vi "SplineHelp_getQuinticSplinesFromControlVectors_ORIG.vi"(11 "ControlVectors":T1[](array[typedef])) -> (0 "error out":errorcluster, 3 "splines":T2[](array[typedef]))   [LabVIEW 2019]
doc: "Returns a set of quintic splines corresponding to the provided control vectors. The user is free to set the direction of all control vectors. Continuous curvature is guaranteed throughout the path.\n\nParameters:\n - controlVectors - The control vectors.\n\nReturns:\n - Splines - A vector of quintic hermite splines that interpolate through the provided waypoints.\n - Error Out - The returned error cluster"
uses:
  SPLINE.ctl
  <vilib>/Analysis/Matrix/Datatypes/RealMatrix.ctl
  SPLINE_CTRL_VECTOR.ctl
  Trajectory_Library.lvlib
  <vilib>/Analysis/Matrix/NI_Matrix.lvlib
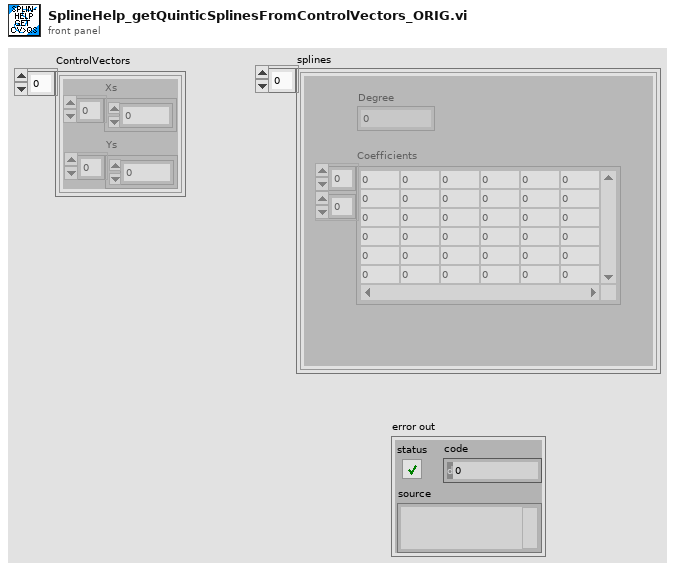
[diagram p1: front panel]
types:
  T1 = typedef "Trajectory_Library.lvlib/SPLINE_CTRL_VECTOR.ctl" = cluster{"Xs":dbl[], "Ys":dbl[]}
  T2 = typedef "Trajectory_Library.lvlib/SPLINE.ctl" = cluster{"Degree":i32, "Coefficients":T3}
  T3 = typedef "NI_Matrix.lvlib/RealMatrix.ctl" = dbl[][]
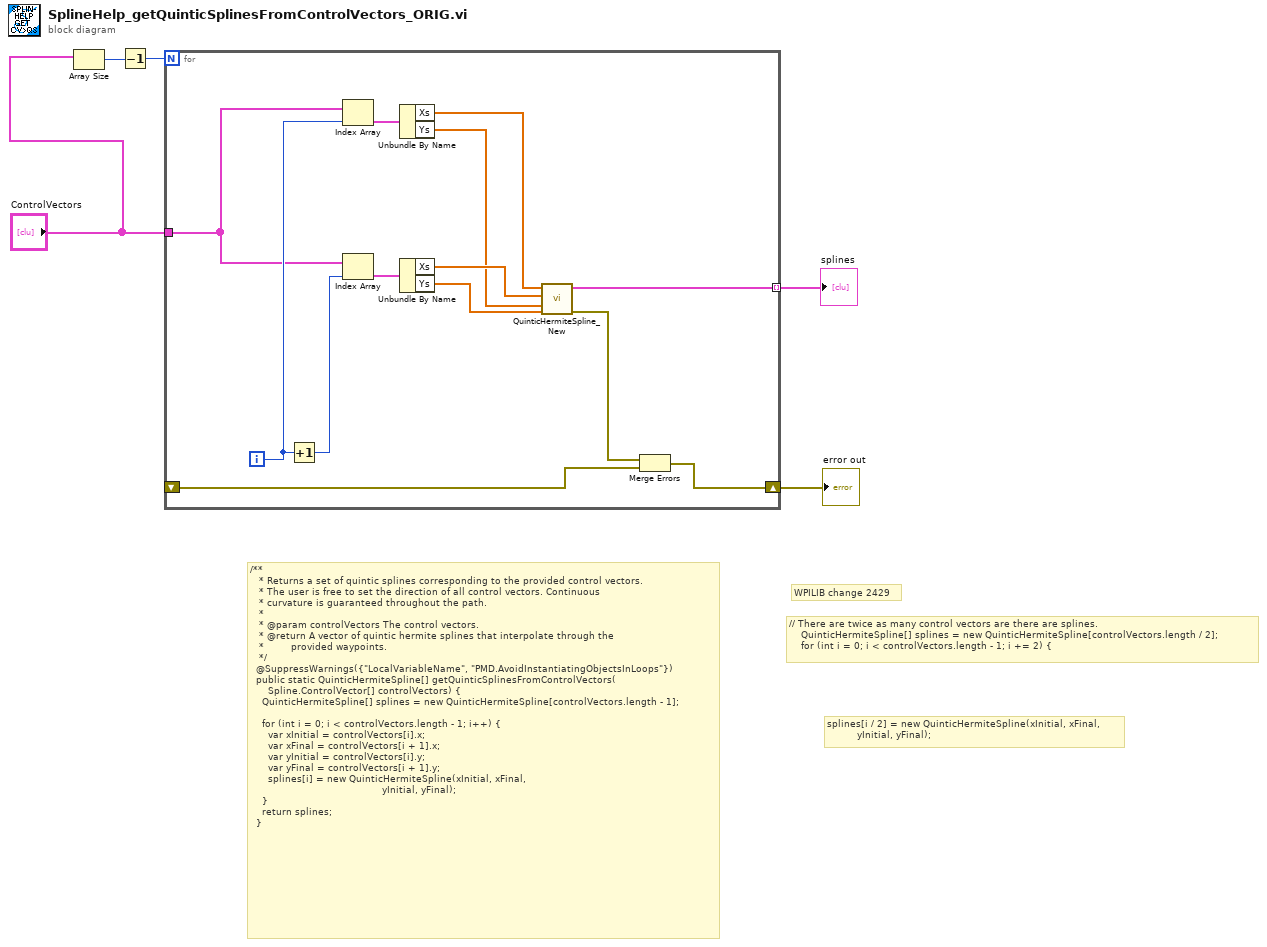
[diagram p0: block diagram]
diagram:
  # "splines[i / 2] = new QuinticHermiteSpline(xInitial, xFinal,\n          yInitial, yFinal);"
  # "WPILIB change 2429"
  # "// There are twice as many control vectors are there are splines.\n    QuinticHermiteSpline[] splines = new QuinticHermiteSpline[controlVectors.length / 2];\n    for (int i = 0; i < controlVectors.length - 1; i += 2) {"
  # "/**\n   * Returns a set of quintic splines corresponding to the provided control vectors.\n   * The user is free to set the direction of all control vectors. Continuous\n   * curvature is guaranteed throughout the path.\n   *\n   * @param controlVectors The control vectors.\n   * @return A vector of quintic hermite splines that interpolate through the\n   *         provided waypoints.\n   */\n  @SuppressWarnings({\"LocalVariableName\", \"PMD.AvoidInstantiatingObjectsInLoops\"})\n  public static QuinticHermiteSpline[] getQuinticSplinesFromControlVectors(\n      Spline.ControlVector[] controlVectors) {\n    QuinticHermiteSpline[] splines = new QuinticHermiteSpline[controlVectors.length - 1];\n\n    for (int i = 0; i < controlVectors.length - 1; i++) {\n      var xInitial = controlVectors[i].x;\n      var xFinal = controlVectors[i + 1].x;\n      var yInitial = controlVectors[i].y;\n      var yFinal = controlVectors[i + 1].y;\n      splines[i] = new QuinticHermiteSpline(xInitial, xFinal,\n                                            yInitial, yFinal);\n    }\n    return splines;\n  }"
  n1 = Array Size(array="ControlVectors") -> (size(s)=w2:i32)
  n2 = Decrement(x=w2) -> (x-1=w3:i32)
  n3 = for {
    N: w3 -> [_]
    tunnel: [w18] -> w5 mode=indexing
    shift-right: [w14] -> w4
    shift-left: _ -> [w15]
    tunnel: "ControlVectors" -> [w12]
    i -> [w17]
    n4 = Increment(x=w17) -> (x+1=w16:i32)
    n5 = Index Array(array=w12, index=w17) -> (element=w11:T1)
    n6 = Index Array(array=w12, index=w16) -> (element=w10:T1)
    n7 = Unbundle By Name(w11) -> ("Xs"=w9:dbl[], "Ys"=w7:dbl[])
    n8 = Unbundle By Name(w10) -> ("Xs"=w8:dbl[], "Ys"=w6:dbl[])
    n9 = call "QuinticHermiteSpline_New.vi"("yFinalCtrlVector"=w6, "yInitialCtrlVector"=w7, "xFinalCtrlVector"=w8, "XInitialCtrlVector"=w9) -> ("error out"=w13:errorcluster, "QuinticHermiteSpline"=w18:T2)  [unwired: 6 in]
    n10 = Merge Errors(w13, w15) -> (w14:errorcluster)
  }
  "error out" <- w4
  "splines" <- w5
